vi "Prepare DB Connect Path (SubVI).vi"(0 "connectString":path, 1 "error in":errorcluster) -> (2 "App.Dir":path, 3 "appended path":path, 4 "error out":errorcluster)   [LabVIEW 2015]
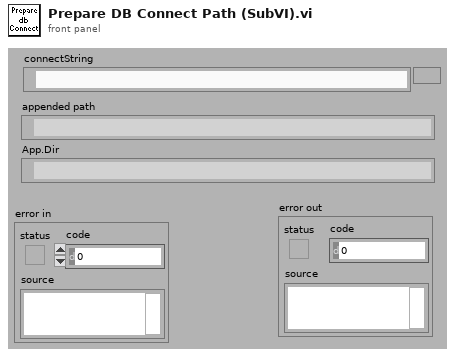
[diagram p1: front panel]
types:
  T1 = enum32{"invalid app kind", "Development System", "Run Time System", "Student Edition", "Embedded LabVIEW", "Evaluation", "Custom"}
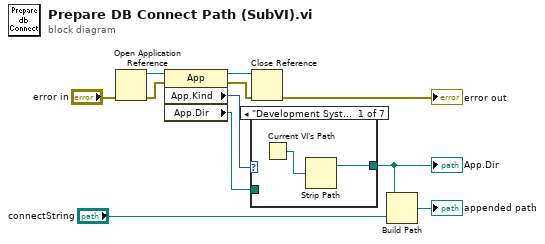
[diagram p0: block diagram]
diagram:
  n1 = Open Application Reference(8:"error in") -> (0:w7:errorcluster, 3:w8:refnum<vi>)  [unwired: 3 out]
  n2 = property class="App"(reference=w8, error in=w7) -> (reference out=w6:refnum<vi>, error out=w5:errorcluster, "App.Kind"=w4:T1, "App.Dir"=w3:path)
  n3 = case shown="\"Development System\"" w4 {
    tunnel: [w12 w14 w15 w16 w17 w18 w19] -> w9
    tunnel: w3 -> [_ w14 w15 w16 w17 w18 w19]
    frame "Development System" {
      n4 = Current VI's Path() -> (path=w13:path)
      n5 = Strip Path(path=w13) -> (stripped path=w12:path)  [unwired: 1 out]
    }
    frame "Run Time System" {
    }
    frame "Student Edition" {
    }
    frame "Embedded LabVIEW" {
    }
    frame "Evaluation" {
    }
    frame "Custom" {
    }
    frame "invalid app kind" {
    }
  }
  "App.Dir" <- w9
  n6 = Close Reference(reference=w6, error in (no error)=w5) -> (error out=→"error out":errorcluster)
  n7 = Build Path(base path=w9, name or relative path="connectString") -> (appended path=→"appended path":path)
